vi "log analysis_gps.vi"() -> ()   [LabVIEW 2019] (continued)
0.4129,0.2981,0.5511,0.1100,0.0931,0.0771,0.1575,0.1588,4.9163,0f000001,0*d9024070\n\t", "INSPVAXA,USB3,0,48.5,FINESTEERING,2107,281880.250,02000000,471d,15824;INS_ALIGNMENT_COMPLETE,INS_RTKFIXED,37.37117348165,126.72305623679,7.9838,22.3000,-0.0959,0.2852,0.0145,-0.523517116,0.173445039,107.625224225,0.4131,0.2981,0.5507,0.1100,0.0932,0.0771,0.1574,0.1588,4.9179,0f000001,0*6bf7a559\n\t", "INSPVAXA,USB3,0,48.5,FINESTEERING,2107,281880.750,02000000,471d,15824;INS_ALIGNMENT_COMPLETE,INS_RTKFIXED,37.37117294431,126.72305789660,7.9831,22.3000,-0.0852,0.2698,0.0141,-0.555772515,0.079408991,107.669635072,0.4131,0.2981,0.5507,0.1100,0.0932,0.0771,0.1574,0.1588,4.9179,0f000001,0*1742ce26\n\t", "INSPVAXA,USB3,0,47.5,FINESTEERING,2107,281881.250,02000000,471d,15824;INS_ALIGNMENT_COMPLETE,INS_RTKFIXED,37.37117244492,126.72305941240,7.9826,22.3000,-0.0757,0.2574,0.0112,-0.499737353,0.074053137,107.349848920,0.4135,0.2983,0.5505,0.1102,0.0933,0.0771,0.1574,0.1588,4.9194,0f000001,0*402f3f2b\n\t", "INSPVAXA,USB3,0,47.5,FINESTEERING,2107,281881.750,02000000,471d,15824;INS_ALIGNMENT_COMPLETE,INS_RTKFIXED,37.37117196738,126.72306091172,7.9831,22.3000,-0.0783,0.2660,0.0186,-0.416436951,0.088853428,106.696307007,0.4135,0.2983,0.5505,0.1102,0.0933,0.0771,0.1574,0.1588,4.9194,0f000001,0*620f9249\n\t", "INSPVAXA,USB3,0,44.5,FINESTEERING,2107,281882.250,02000000,471d,15824;INS_ALIGNMENT_COMPLETE,INS_RTKFIXED,37.37117150853,126.72306241559,7.9850,22.3000,-0.0608,0.2451,0.0066,-0.406550409,0.024677772,105.806071956,0.4138,0.2984,0.5505,0.1102,0.0933,0.0771,0.1573,0.1588,4.9208,0f000001,0*20d266fd\n\t", "INSPVAXA,USB3,0,46.5,FINESTEERING,2107,281883.250,02000000,471d,15824;INS_ALIGNMENT_COMPLETE,INS_RTKFIXED,37.37117067641,126.72306545358,7.9876,22.3000,-0.0777,0.2473,0.0004,-0.446761173,0.141959315,103.301752998,0.4139,0.2985,0.5503,0.1102,0.0932,0.0771,0.1572,0.1587,4.9224,0f000001,0*34b690f3\n\t", "INSPVAXA,USB3,0,46.5,FINESTEERING,2107,281883.750,02000000,471d,15824;INS_ALIGNMENT_COMPLETE,INS_RTKFIXED,37.37117030441,126.72306700472,7.9899,22.3000,-0.0617,0.2696,0.0265,-0.542142026,0.246764373,102.057621753,0.4139,0.2985,0.5503,0.1102,0.0932,0.0771,0.1572,0.1587,4.9224,0f000001,0*016cab57\n\t", "INSPVAXA,USB3,0,48.0,FINESTEERING,2107,281884.750,02000000,471d,15824;INS_ALIGNMENT_COMPLETE,INS_RTKFIXED,37.37116962918,126.72307017450,7.9972,22.3000,-0.0537,0.2746,0.0133,-0.660873018,0.326948339,100.072587895,0.4139,0.2985,0.5502,0.1101,0.0931,0.0771,0.1571,0.1587,4.9240,0f000001,0*1475196f\n\t", "INSPVAXA,USB3,0,46.5,FINESTEERING,2107,281885.250,02000000,471d,15824;INS_ALIGNMENT_COMPLETE,INS_RTKFIXED,37.37116932974,126.72307175980,8.0003,22.3000,-0.0553,0.2834,0.0118,-0.680106492,0.432078155,99.489485657,0.4137,0.2985,0.5500,0.1099,0.0931,0.0771,0.1571,0.1587,4.9256,0f000001,0*384d6b59\n\t", "INSPVAXA,USB3,0,48.5,FINESTEERING,2107,281886.250,02000000,471d,15824;INS_ALIGNMENT_COMPLETE,INS_RTKFIXED,37.37116876559,126.72307497858,8.0043,22.3000,-0.0505,0.2700,0.0197,-0.630737523,0.236103622,98.774518000,0.4135,0.2984,0.5500,0.1099,0.0931,0.0771,0.1570,0.1587,4.9269,0f000001,0*06e1d073\n\t", "INSPVAXA,USB3,0,48.5,FINESTEERING,2107,281886.750,02000000,471d,15824;INS_ALIGNMENT_COMPLETE,INS_RTKFIXED,37.37116849518,126.72307655860,8.0058,22.3000,-0.0479,0.2894,0.0098,-0.729843639,0.253785173,98.685149837,0.4135,0.2984,0.5500,0.1099,0.0931,0.0771,0.1570,0.1587,4.9269,0f000001,0*6ed17162\n\t", "INSPVAXA,USB3,0,47.5,FINESTEERING,2107,281887.750,02000000,471d,15824;INS_ALIGNMENT_COMPLETE,INS_RTKFIXED,37.37116794085,126.72307975608,8.0103,22.3000,-0.0483,0.2817,0.0113,-0.853841864,0.188447476,98.810925200,0.4129,0.2983,0.5497,0.1100,0.0933,0.0771,0.1570,0.1587,4.9280,0f000001,0*b49a26d4\n\t", "INSPVAXA,USB3,0,50.0,FINESTEERING,2107,281888.250,02000000,471d,15824;INS_ALIGNMENT_COMPLETE,INS_RTKFIXED,37.37116766545,126.72308132013,8.0114,22.3000,-0.0457,0.2739,0.0034,-0.968854092,0.193025151,98.915996054,0.4125,0.2983,0.5497,0.1101,0.0935,0.0771,0.1571,0.1587,4.9288,0f000001,0*9b5c7e2f\n\t", "INSPVAXA,USB3,0,44.5,FINESTEERING,2107,281889.750,02000000,471d,15824;INS_ALIGNMENT_COMPLETE,INS_RTKFIXED,37.37116676559,126.72308604479,8.0182,22.3000,-0.0625,0.3054,0.0209,-0.972087805,-0.015873358,99.423505279,0.4122,0.2983,0.5496,0.1103,0.0935,0.0771,0.1571,0.1586,4.9293,0f000001,0*71ed46ba\n\t", "INSPVAXA,USB3,0,49.0,FINESTEERING,2107,281892.250,02000000,471d,15824;INS_ALIGNMENT_COMPLETE,INS_RTKFIXED,37.37116500965,126.72309429685,8.0266,22.3000,-0.0800,0.3032,0.0106,-1.000045816,-0.250485086,101.581647169,0.4117,0.2986,0.5496,0.1105,0.0935,0.0771,0.1571,0.1583,4.9290,0f000001,0*ebccc2b7\n\t", "INSPVAXA,USB3,0,49.0,FINESTEERING,2107,281892.750,02000000,471d,15824;INS_ALIGNMENT_COMPLETE,INS_RTKFIXED,37.37116464489,126.72309588370,8.0261,22.3000,-0.0746,0.2919,0.0013,-0.966505403,-0.074133262,102.355415882,0.4117,0.2986,0.5496,0.1105,0.0935,0.0771,0.1571,0.1583,4.9290,0f000001,0*e99d934b\n\t", "INSPVAXA,USB3,0,46.0,FINESTEERING,2107,281893.750,02000000,471d,15824;INS_ALIGNMENT_COMPLETE,INS_RTKFIXED,37.37116386545,126.72309901774,8.0239,22.3000,-0.0747,0.2810,0.0135,-0.903776454,0.116604665,103.770415844,0.4122,0.2987,0.5500,0.1103,0.0933,0.0771,0.1570,0.1582,4.9290,0f000001,0*419476b1\n\t", "INSPVAXA,USB3,0,46.0,FINESTEERING,2107,281895.250,02000000,471d,15824;INS_ALIGNMENT_COMPLETE,INS_RTKFIXED,37.37116255070,126.72310371548,8.0235,22.3000,-0.0988,0.2868,0.0058,-0.574989155,-0.045458111,105.108744593,0.4125,0.2988,0.5503,0.1099,0.0932,0.0771,0.1569,0.1580,4.9303,0f000001,0*d88c0d09\n\t", "INSPVAXA,USB3,0,48.5,FINESTEERING,2107,281911.800,02000000,471d,15824;INS_ALIGNMENT_COMPLETE,INS_RTKFIXED,37.37115003469,126.72315448526,8.0928,22.3000,-0.0862,0.2747,0.0289,-0.974037724,0.304621853,104.802649899,0.4114,0.2983,0.5457,0.1097,0.0931,0.0770,0.1565,0.1577,4.9486,0f000001,0*2c2c9bcb\n\t", "INSPVAXA,USB3,0,44.5,FINESTEERING,2107,281916.300,02000000,471d,15824;INS_ALIGNMENT_COMPLETE,INS_RTKFIXED,37.37114589383,126.72316794464,8.1130,22.3000,-0.1148,0.2616,0.0217,-1.148454264,0.358744068,107.173500933,0.4066,0.2960,0.5376,0.1089,0.0926,0.0764,0.1563,0.1575,4.9560,0f000001,0*04915923\n\t", "INSPVAXA,USB3,0,45.5,FINESTEERING,2107,281917.300,02000000,471d,15824;INS_ALIGNMENT_COMPLETE,INS_RTKFIXED,37.37114488879,126.72317107328,8.1169,22.3000,-0.1215,0.2812,0.0224,-1.106333570,0.024690310,107.280249927,0.4087,0.2971,0.5398,0.1096,0.0930,0.0767,0.1563,0.1576,4.9575,0f000001,0*9d9688b2\n\t", "INSPVAXA,USB3,0,48.5,FINESTEERING,2107,281918.800,02000000,471d,15824;INS_ALIGNMENT_COMPLETE,INS_RTKFIXED,37.37114346070,126.72317566723,8.1280,22.3000,-0.1055,0.2660,0.0189,-1.458385155,0.133384448,106.568583790,0.4097,0.2978,0.5415,0.1097,0.0931,0.0768,0.1562,0.1576,4.9589,0f000001,0*d5a698ac\n\t", "INSPVAXA,USB3,0,44.0,FINESTEERING,2107,281920.800,02000000,471d,15824;INS_ALIGNMENT_COMPLETE,INS_RTKFIXED,37.37114173890,126.72318175372,8.1382,22.3000,-0.1108,0.2593,0.0206,-1.441924072,0.214033238,104.164659813,0.4062,0.2959,0.5371,0.1088,0.0925,0.0764,0.1560,0.1575,4.9615,0f000001,0*96e1255f\n\t", "INSPVAXA,USB3,0,48.0,FINESTEERING,2107,281922.800,02000000,471d,15824;INS_ALIGNMENT_COMPLETE,INS_RTKFIXED,37.37114021696,126.72318792765,8.1435,22.3000,-0.0885,0.2559,0.0232,-1.379339371,0.280141219,102.369247536,0.4099,0.2977,0.5413,0.1094,0.0930,0.0768,0.1560,0.1575,4.9637,0f000001,0*69df9f1e\n\t", "INSPVAXA,USB3,0,48.0,FINESTEERING,2107,281923.800,02000000,471d,15824;INS_ALIGNMENT_COMPLETE,INS_RTKFIXED,37.37113946532,126.72319101111,8.1415,22.3000,-0.0919,0.2757,0.0244,-1.061632800,0.175078722,102.246819670,0.4052,0.2954,0.5349,0.1085,0.0923,0.0763,0.1558,0.1574,4.9646,0f000001,0*a7ce5637\n\t", "INSPVAXA,USB3,0,47.5,FINESTEERING,2107,281924.300,02000000,471d,15824;INS_ALIGNMENT_COMPLETE,INS_RTKFIXED,37.37113911142,126.72319252846,8.1410,22.3000,-0.0952,0.2671,0.0232,-1.111033615,0.347415537,102.293993552,0.4024,0.2943,0.5302,0.1081,0.0921,0.0760,0.1558,0.1574,4.9658,0f000001,0*38544010\n\t", "INSPVAXA,USB3,0,45.0,FINESTEERING,2107,281925.300,02000000,471d,15824;INS_ALIGNMENT_COMPLETE,INS_RTKFIXED,37.37113840523,126.72319556014,8.1418,22.3000,-0.0995,0.2785,0.0107,-1.061115952,0.585903196,102.432927019,0.4060,0.2962,0.5334,0.1089,0.0927,0.0764,0.1559,0.1575,4.9673,0f000001,0*3a408327\n\t", "INSPVAXA,USB3,0,47.0,FINESTEERING,2107,281926.800,02000000,471d,15824;INS_ALIGNMENT_COMPLETE,INS_RTKFIXED,37.37113727918,126.72320023038,8.1455,22.3000,-0.1010,0.2911,0.0183,-0.984134489,0.435250920,102.983735265,0.4086,0.2974,0.5364,0.1094,0.0930,0.0766,0.1559,0.1575,4.9689,0f000001,0*added2fa\n\t", "INSPVAXA,USB3,0,47.0,FINESTEERING,2107,281927.300,02000000,471d,15824;INS_ALIGNMENT_COMPLETE,INS_RTKFIXED,37.37113689419,126.72320185554,8.1485,22.3000,-0.1162,0.2988,0.0149,-1.006289928,0.413812859,103.207528579,0.4104,0.2981,0.5392,0.1096,0.0931,0.0768,0.1559,0.1575,4.9705,0f000001,0*f16ca07f\n\t", "INSPVAXA,USB3,0,48.5,FINESTEERING,2107,281928.300,02000000,471d,15824;INS_ALIGNMENT_COMPLETE,INS_RTKFIXED,37.37113611712,126.72320505771,8.1519,22.3000,-0.1090,0.2747,0.0204,-1.003980173,0.404401271,103.811290655,0.4113,0.2984,0.5414,0.1096,0.0931,0.0769,0.1559,0.1574,4.9721,0f000001,0*ce8a0efc\n\t", "INSPVAXA,USB3,0,47.0,FINESTEERING,2107,281929.300,02000000,471d,15824;INS_ALIGNMENT_COMPLETE,INS_RTKFIXED,37.37113535023,126.72320815380,8.1534,22.3000,-0.0933,0.2709,0.0146,-1.164082323,0.102490422,104.875233542,0.4118,0.2986,0.5433,0.1096,0.0930,0.0770,0.1559,0.1574,4.9735,0f000001,0*94f0b5d4\n\t", "INSPVAXA,USB3,0,49.0,FINESTEERING,2107,281930.300,02000000,471d,15824;INS_ALIGNMENT_COMPLETE,INS_RTKFIXED,37.37113452225,126.72321122959,8.1544,22.3000,-0.0922,0.2630,0.0022,-1.151432888,0.140260407,106.440387814,0.4107,0.2981,0.5430,0.1094,0.0928,0.0769,0.1559,0.1573,4.9747,0f000001,0*0b618f55\n\t", "INSPVAXA,USB3,0,46.5,FINESTEERING,2107,281931.300,02000000,471d,15824;INS_ALIGNMENT_COMPLETE,INS_RTKFIXED,37.37113361810,126.72321422448,8.1520,22.3000,-0.1052,0.2573,0.0056,-1.026339902,0.274196380,108.020288204,0.4094,0.2975,0.5419,0.1091,0.0927,0.0767,0.1558,0.1572,4.9758,0f000001,0*a4843e8d\n\t", "INSPVAXA,USB3,0,46.5,FINESTEERING,2107,281931.800,02000000,471d,15824;INS_ALIGNMENT_COMPLETE,INS_RTKFIXED,37.37113315554,126.72321571726,8.1497,22.3000,-0.1071,0.2546,0.0196,-1.189773358,0.228457398,108.723422614,0.4094,0.2975,0.5419,0.1091,0.0927,0.0767,0.1558,0.1572,4.9758,0f000001,0*2e0e4421\n\t", "INSPVAXA,USB3,0,46.5,FINESTEERING,2107,281932.800,02000000,471d,15824;INS_ALIGNMENT_COMPLETE,INS_RTKFIXED,37.37113218049,126.72321869652,8.1511,22.3000,-0.1122,0.2507,0.0244,-0.970343448,0.146977674,109.553158017,0.4088,0.2971,0.5408,0.1090,0.0926,0.0766,0.1558,0.1571,4.9770,0f000001,0*3507ce24\n\t", "INSPVAXA,USB3,0,46.5,FINESTEERING,2107,281933.300,02000000,471d,15824;INS_ALIGNMENT_COMPLETE,INS_RTKFIXED,37.37113167702,126.72322018624,8.1496,22.3000,-0.1082,0.2476,0.0112,-0.825942181,0.095830764,109.777034035,0.4078,0.2967,0.5396,0.1089,0.0928,0.0765,0.1558,0.1571,4.9781,0f000001,0*1bc6ffe3\n\t", "INSPVAXA,USB3,0,48.5,FINESTEERING,2107,281934.800,02000000,471d,15824;INS_ALIGNMENT_COMPLETE,INS_RTKFIXED,37.37113025084,126.72322449049,8.1432,22.3000,-0.1047,0.2449,0.0092,-0.950644980,-0.057069061,110.390138086,0.4095,0.2975,0.5414,0.1094,0.0930,0.0767,0.1558,0.1572,4.9791,0f000001,0*563aefdc\n\t", "INSPVAXA,USB3,0,46.5,FINESTEERING,2107,281935.300,02000000,471d,15824;INS_ALIGNMENT_COMPLETE,INS_RTKFIXED,37.37112977302,126.72322590337,8.1419,22.3000,-0.1049,0.2498,0.0104,-0.942926672,-0.039965742,110.562621563,0.4110,0.2981,0.5430,0.1097,0.0932,0.0768,0.1557,0.1572,4.9802,0f000001,0*75823065\n\t", "INSPVAXA,USB3,0,46.5,FINESTEERING,2107,281935.800,02000000,471d,15824;INS_ALIGNMENT_COMPLETE,INS_RTKFIXED,37.37112927929,126.72322735116,8.1404,22.3000,-0.1170,0.2611,0.0107,-1.050315231,0.030356412,110.657182537,0.4110,0.2981,0.5430,0.1097,0.0932,0.0768,0.1557,0.1572,4.9802,0f000001,0*518b09cb\n\t", "INSPVAXA,USB3,0,46.5,FINESTEERING,2107,281936.800,02000000,471d,15824;INS_ALIGNMENT_COMPLETE,INS_RTKFIXED,37.37112820521,126.72323038225,8.1394,22.3000,-0.1018,0.2637,0.0146,-1.057508289,0.307807352,110.761201411,0.4116,0.2984,0.5442,0.1099,0.0933,0.0768,0.1556,0.1572,4.9813,0f000001,0*af3d1803\n\t", "INSPVAXA,USB3,0,50.5,FINESTEERING,2107,281937.300,02000000,471d,15824;INS_ALIGNMENT_COMPLETE,INS_RTKFIXED,37.37112766751,126.72323189029,8.1401,22.3000,-0.1026,0.2581,0.0148,-1.068160739,0.434910636,110.781904334,0.4120,0.2986,0.5450,0.1099,0.0934,0.0769,0.1555,0.1571,4.9826,0f000001,0*c1896a38\n\t", "INSPVAXA,USB3,0,50.5,FINESTEERING,2107,281937.800,02000000,471d,15824;INS_ALIGNMENT_COMPLETE,INS_RTKFIXED,37.37112712976,126.72323340459,8.1402,22.3000,-0.1084,0.2649,0.0122,-1.080841395,0.445033455,110.675623077,0.4120,0.2986,0.5450,0.1099,0.0934,0.0769,0.1555,0.1571,4.9826,0f000001,0*491a3d94\n\t", "INSPVAXA,USB3,0,48.0,FINESTEERING,2107,281938.300,02000000,471d,15824;INS_ALIGNMENT_COMPLETE,INS_RTKFIXED,37.37112660699,126.72323489042,8.1401,22.3000,-0.1000,0.2525,0.0063,-1.085397063,0.578788009,110.287744750,0.4123,0.2988,0.5457,0.1100,0.0934,0.0769,0.1554,0.1571,4.9841,0f000001,0*2d3bbc15\n\t", "INSPVAXA,USB3,0,48.0,FINESTEERING,2107,281939.300,02000000,471d,15824;INS_ALIGNMENT_COMPLETE,INS_RTKFIXED,37.37112559001,126.72323792632,8.1403,22.3000,-0.1055,0.2758,-0.0006,-1.140987181,0.421010815,109.156991260,0.4088,0.2970,0.5408,0.1093,0.0930,0.0765,0.1552,0.1570,4.9858,0f000001,0*79dbeeff\n\t", "INSPVAXA,USB3,0,48.0,FINESTEERING,2107,281939.800,02000000,471d,15824;INS_ALIGNMENT_COMPLETE,INS_RTKFIXED,37.37112510387,126.72323945796,8.1419,22.3000,-0.1142,0.2830,0.0009,-1.038854179,0.260898620,108.398784803,0.4088,0.2970,0.5408,0.1093,0.0930,0.0765,0.1552,0.1570,4.9858,0f000001,0*5c0fede7\n\t", "INSPVAXA,USB3,0,46.0,FINESTEERING,2107,281940.800,02000000,471d,15824;INS_ALIGNMENT_COMPLETE,INS_RTKFIXED,37.37112421905,126.72324251509,8.1454,22.3000,-0.0917,0.2666,0.0165,-1.172718018,0.154583704,106.881501399,0.4059,0.2957,0.5358,0.1088,0.0926,0.0762,0.1550,0.1569,4.9872,0f000001,0*d9c0846d\n\t", "INSPVAXA,USB3,0,46.0,FINESTEERING,2107,281941.300,02000000,471d,15824;INS_ALIGNMENT_COMPLETE,INS_RTKFIXED,37.37112376695,126.72324410387,8.1465,22.3000,-0.0867,0.2640,0.0120,-1.227884261,0.058014022,106.288086050,0.4040,0.2951,0.5320,0.1086,0.0925,0.0760,0.1549,0.1568,4.9885,0f000001,0*dacbaea6\n\t", "INSPVAXA,USB3,0,46.0,FINESTEERING,2107,281941.800,02000000,471d,15824;INS_ALIGNMENT_COMPLETE,INS_RTKFIXED,37.37112332750,126.72324562221,8.1480,22.3000,-0.0872,0.2775,0.0087,-1.185427443,0.271965385,105.771989381,0.4040,0.2951,0.5320,0.1086,0.0925,0.0760,0.1549,0.1568,4.9885,0f000001,0*6fc02a4a\n\t", "INSPVAXA,USB3,0,48.0,FINESTEERING,2107,281942.300,02000000,471d,15824;INS_ALIGNMENT_COMPLETE,INS_RTKFIXED,37.37112291228,126.72324712545,8.1496,22.3000,-0.0882,0.2861,0.0099,-1.302160534,0.485080521,105.427907916,0.4030,0.2950,0.5294,0.1085,0.0925,0.0759,0.1549,0.1568,4.9897,0f000001,0*226a6453\n\t", "INSPVAXA,USB3,0,48.0,FINESTEERING,2107,281942.800,02000000,471d,15824;INS_ALIGNMENT_COMPLETE,INS_RTKFIXED,37.37112248759,126.72324869742,8.1506,22.3000,-0.0906,0.2829,0.0087,-1.416858091,0.320755573,105.114795692,0.4030,0.2950,0.5294,0.1085,0.0925,0.0759,0.1549,0.1568,4.9897,0f000001,0*d431e262\n\t", "DUALANTENNAHEADINGA,USB3,0,49.0,FINESTEERING,2107,281943.300,02000000,d426,15824;SOL_COMPUTED,NARROW_FLOAT,-1.000000000,117.129844666,-65.553436279,0.0,360.000000000,180.000000000,\"631T\",17,7,7,7,04,00,20,03*a0d5c722\n\t", "INSPVAXA,USB3,0,49.0,FINESTEERING,2107,281943.800,02000000,471d,15824;INS_ALIGNMENT_COMPLETE,INS_RTKFIXED,37.37112165725,126.72325176425,8.1526,22.3000,-0.0982,0.2663,0.0142,-1.467433834,0.522949098,104.939300217,0.4063,0.2966,0.5325,0.1091,0.0930,0.0763,0.1549,0.1569,4.9906,0f000001,0*8fab3056\n\t", "INSPVAXA,USB3,0,49.0,FINESTEERING,2107,281944.300,02000000,471d,15824;INS_ALIGNMENT_COMPLETE,INS_RTKFIXED,37.37112121835,126.72325329902,8.1549,22.3000,-0.0986,0.2706,0.0194,-1.288520157,0.440494920,104.991020886,0.4098,0.2978,0.5362,0.1096,0.0931,0.0766,0.1549,0.1570,4.9912,0f000001,0*9299408f\n\t", "INSPVAXA,USB3,0,49.0,FINESTEERING,2107,281944.800,02000000,471d,15824;INS_ALIGNMENT_COMPLETE,INS_RTKFIXED,37.37112078350,126.72325484675,8.1574,22.3000,-0.0973,0.2817,0.0195,-1.314361795,0.302961739,105.060294350,0.4098,0.2978,0.5362,0.1096,0.0931,0.0766,0.1549,0.1570,4.9912,0f000001,0*74de03e1\n\t", "INSPVAXA,USB3,0,50.5,FINESTEERING,2107,281945.300,02000000,471d,15824;INS_ALIGNMENT_COMPLETE,INS_RTKFIXED,37.37112035973,126.72325634532,8.1592,22.3000,-0.0947,0.2865,0.0177,-1.337666761,0.342742337,105.119539475,0.4078,0.2967,0.5345,0.1091,0.0927,0.0765,0.1549,0.1569,4.9918,0f000001,0*40c63c80\n\t", "DUALANTENNAHEADINGA,USB3,0,50.5,FINESTEERING,2107,281945.800,02000000,d426,15824;SOL_COMPUTED,NARROW_FLOAT,-1.000000000,110.210548401,-43.006103516,0.0,360.000000000,180.000000000,\"631T\",17,7,7,7,04,00,20,03*d65a3eb4\n\t", "DUALANTENNAHEADINGA,USB3,0,50.5,FINESTEERING,2107,281946.300,02000000,d426,15824;SOL_COMPUTED,NARROW_FLOAT,-1.000000000,136.716491699,-61.625274658,0.0,360.000000000,180.000000000,\"631T\",17,7,7,7,04,00,20,03*380a706b\n\t", "INSPVAXA,USB3,0,50.5,FINESTEERING,2107,281946.800,02000000,471d,15824;INS_ALIGNMENT_COMPLETE,INS_RTKFIXED,37.37111906801,126.72326090690,8.1646,22.3000,-0.0999,0.2885,0.0123,-1.416267608,0.329165481,105.354050291,0.4059,0.2956,0.5320,0.1087,0.0926,0.0762,0.1548,0.1568,4.9924,0f000001,0*28d47c8b\n\t", "INSPVAXA,USB3,0,45.5,FINESTEERING,2107,281947.300,02000000,471d,15824;INS_ALIGNMENT_COMPLETE,INS_RTKFIXED,37.37111863332,126.72326240814,8.1666,22.3000,-0.0961,0.2751,0.0203,-1.384816441,0.416422862,105.503918541,0.4041,0.2951,0.5298,0.1085,0.0924,0.0761,0.1549,0.1568,4.9930,0f000001,0*a10fe9f6\n\t", "INSPVAXA,USB3,0,45.5,FINESTEERING,2107,281947.800,02000000,471d,15824;INS_ALIGNMENT_COMPLETE,INS_RTKFIXED,37.37111818250,126.72326395318,8.1681,22.3000,-0.0954,0.2801,0.0190,-1.275593165,0.401297013,105.699844035,0.4041,0.2951,0.5298,0.1085,0.0924,0.0761,0.1549,0.1568,4.9930,0f000001,0*107534c5\n\t", "INSPVAXA,USB3,0,45.5,FINESTEERING,2107,281948.300,02000000,471d,15824;INS_ALIGNMENT_COMPLETE,INS_RTKFIXED,37.37111773045,126.72326549713,8.1704,22.3000,-0.0978,0.2931,0.0097,-1.304299318,0.393717319,105.933712093,0.4025,0.2945,0.5274,0.1083,0.0923,0.0760,0.1549,0.1567,4.9937,0f000001,0*f7f3e128\n\t", "DUALANTENNAHEADINGA,USB3,0,45.5,FINESTEERING,2107,281948.800,02000000,d426,15824;SOL_COMPUTED,NARROW_FLOAT,-1.000000000,181.763427734,-33.084808350,0.0,210.189346313,180.000000000,\"631T\",18,7,7,7,04,00,20,03*dd4d4ec1\n\t", "INSPVAXA,USB3,0,49.0,FINESTEERING,2107,281949.300,02000000,471d,15824;INS_ALIGNMENT_COMPLETE,INS_RTKFIXED,37.37111680262,126.72326852511,8.1763,22.3000,-0.0970,0.2807,0.0172,-1.183781176,0.416069138,106.325153596,0.4018,0.2942,0.5256,0.1083,0.0923,0.0759,0.1549,0.1566,4.9947,0f000001,0*47cb080a\n\t", "INSPVAXA,USB3,0,49.0,FINESTEERING,2107,281949.800,02000000,471d,15824;INS_ALIGNMENT_COMPLETE,INS_RTKFIXED,37.37111632001,126.72327008687,8.1784,22.3000,-0.0963,0.2886,0.0125,-1.143678600,0.359831061,106.512743553,0.4018,0.2942,0.5256,0.1083,0.0923,0.0759,0.1549,0.1566,4.9947,0f000001,0*07f750f1\n\t", "INSPVAXA,USB3,0,50.0,FINESTEERING,2107,281950.300,02000000,471d,15824;INS_ALIGNMENT_COMPLETE,INS_RTKFIXED,37.37111586312,126.72327158284,8.1822,22.3000,-0.0965,0.2844,0.0140,-1.158757889,0.473761966,106.723274256,0.4019,0.2945,0.5251,0.1083,0.0924,0.0759,0.1549,0.1566,4.9959,0f000001,0*c4604f56\n\t", "INSPVAXA,USB3,0,50.0,FINESTEERING,2107,281950.800,02000000,471d,15824;INS_ALIGNMENT_COMPLETE,INS_RTKFIXED,37.37111539537,126.72327311489,8.1870,22.3000,-0.0882,0.2799,0.0131,-1.063577950,0.631384742,106.921378709,0.4019,0.2945,0.5251,0.1083,0.0924,0.0759,0.1549,0.1566,4.9959,0f000001,0*182037fa\n\t", "DUALANTENNAHEADINGA,USB3,0,50.0,FINESTEERING,2107,281951.300,02000000,d426,15824;SOL_COMPUTED,NARROW_FLOAT,-1.000000000,139.470138550,7.252925396,0.0,360.000000000,180.000000000,\"631T\",16,7,7,7,04,00,20,03*6d09da6c\n\t", "INSPVAXA,USB3,0,50.0,FINESTEERING,2107,281951.800,02000000,471d,15824;INS_ALIGNMENT_COMPLETE,INS_RTKFIXED,37.37111448325,126.72327615215,8.1961,22.3000,-0.0961,0.2823,0.0155,-1.049815385,0.768292718,107.282719412,0.4015,0.2942,0.5235,0.1082,0.0922,0.0758,0.1549,0.1565,4.9974,0f000001,0*bdafe358\n\t", "INSPVAXA,USB3,0,49.0,FINESTEERING,2107,281952.300,02000000,471d,15824;INS_ALIGNMENT_COMPLETE,INS_RTKFIXED,37.37111402480,126.72327764482,8.2001,22.3000,-0.0943,0.2854,0.0221,-1.074547440,0.687119581,107.404842007,0.4042,0.2955,0.5263,0.1087,0.0925,0.0761,0.1549,0.1565,4.9990,0f000001,0*5102a955\n\t", "INSPVAXA,USB3,0,49.0,FINESTEERING,2107,281952.800,02000000,471d,15824;INS_ALIGNMENT_COMPLETE,INS_RTKFIXED,37.37111356857,126.72327910492,8.2050,22.3000,-0.0959,0.2790,0.0249,-1.146713469,0.626149533,107.488269865,0.4042,0.2955,0.5263,0.1087,0.0925,0.0761,0.1549,0.1565,4.9990,0f000001,0*a4159e63\n\t", "DUALANTENNAHEADINGA,USB3,0,51.5,FINESTEERING,2107,281953.300,02000000,d426,15824;SOL_COMPUTED,NARROW_FLOAT,-1.000000000,139.308395386,-63.930755615,0.0,360.000000000,171.725708008,\"631T\",19,7,7,7,04,00,20,03*aebc5255\n\t", "DUALANTENNAHEADINGA,USB3,0,51.5,FINESTEERING,2107,281953.800,02000000,d426,15824;SOL_COMPUTED,NARROW_FLOAT,-1.000000000,139.742797852,-63.902252197,0.0,360.000000000,171.789428711,\"631T\",17,7,7,7,04,00,20,03*2ba0ac3f\n\t", "INSPVAXA,USB3,0,49.5,FINESTEERING,2107,281954.300,02000000,471d,15824;INS_ALIGNMENT_COMPLETE,INS_RTKFIXED,37.37111212186,126.72328367661,8.2114,22.3000,-0.1061,0.2807,0.0084,-1.239615832,0.473328894,107.695107269,0.4028,0.2947,0.5241,0.1082,0.0921,0.0759,0.1549,0.1563,5.0021,0f000001,0*b68b8e11\n\t", "DUALANTENNAHEADINGA,USB3,0,49.5,FINESTEERING,2107,281954.800,02000000,d426,15824;SOL_COMPUTED,NARROW_FLOAT,-1.000000000,123.390388489,-57.995361328,0.0,360.000000000,180.000000000,\"631T\",16,7,7,7,04,00,20,03*cd5e4259\n\t", "DUALANTENNAHEADINGA,USB3,0,47.0,FINESTEERING,2107,281955.300,02000000,d426,15824;SOL_COMPUTED,NARROW_FLOAT,-1.000000000,132.237213135,-56.367187500,0.0,360.000000000,180.000000000,\"631T\",16,7,7,7,04,00,20,03*7928331b\n\t", "DUALANTENNAHEADINGA,USB3,0,47.0,FINESTEERING,2107,281955.800,02000000,d426,15824;SOL_COMPUTED,NARROW_FLOAT,-1.000000000,131.490509033,-56.782928467,0.0,360.000000000,180.000000000,\"631T\",17,7,7,7,04,00,20,03*bed209ba\n\t", "DUALANTENNAHEADINGA,USB3,0,47.0,FINESTEERING,2107,281956.300,02000000,d426,15824;SOL_COMPUTED,NARROW_FLOAT,-1.000000000,120.002708435,27.323427200,0.0,360.000000000,180.000000000,\"631T\",18,7,7,7,04,00,20,03*7e70b057\n\t", "INSPVAXA,USB3,0,47.0,FINESTEERING,2107,281956.800,02000000,471d,15824;INS_ALIGNMENT_COMPLETE,INS_RTKFIXED,37.37110977016,126.72329115727,8.2173,22.3000,-0.1059,0.2673,0.0082,-1.256961721,0.075845968,107.131843549,0.4006,0.2939,0.5214,0.1078,0.0919,0.0757,0.1548,0.1562,5.0048,0f000001,0*c3de906c\n\t", "INSPVAXA,USB3,0,49.0,FINESTEERING,2107,281957.300,02008000,471d,15824;INS_ALIGNMENT_COMPLETE,INS_RTKFIXED,37.37110932178,126.72329265930,8.2173,22.3000,-0.1030,0.2706,0.0074,-1.272872936,0.072348347,106.750132091,0.4007,0.2939,0.5208,0.1079,0.0919,0.0757,0.1548,0.1562,5.0062,0f000001,0*240beb48\n\t", "DUALANTENNAHEADINGA,USB3,0,49.0,FINESTEERING,2107,281957.800,02008000,d426,15824;SOL_COMPUTED,NARROW_FLOAT,-1.000000000,114.580795288,38.922153473,0.0,360.000000000,180.000000000,\"631T\",20,7,7,7,04,00,20,03*611330d6\n\t", "DUALANTENNAHEADINGA,USB3,0,49.5,FINESTEERING,2107,281958.300,02008000,d426,15824;SOL_COMPUTED,NARROW_FLOAT,-1.000000000,104.400451660,-50.100708008,0.0,360.000000000,180.000000000,\"631T\",21,7,7,7,04,00,20,03*9c19a85a\n\t", "DUALANTENNAHEADINGA,USB3,0,49.5,FINESTEERING,2107,281958.800,02008000,d426,15824;SOL_COMPUTED,NARROW_FLOAT,-1.000000000,106.192443848,-50.461669922,0.0,360.000000000,180.000000000,\"631T\",18,7,7,7,04,00,20,03*bd2737c2\n\t", "DUALANTENNAHEADINGA,USB3,0,47.5,FINESTEERING,2107,281959.300,02008000,d426,15824;SOL_COMPUTED,NARROW_FLOAT,-1.000000000,102.626930237,-53.845886230,0.0,360.000000000,180.000000000,\"631T\",18,7,7,7,04,00,20,03*cccf90f6\n\t", "DUALANTENNAHEADINGA,USB3,0,47.5,FINESTEERING,2107,281959.800,02008000,d426,15824;SOL_COMPUTED,NARROW_FLOAT,-1.000000000,103.518684387,-53.796081543,0.0,360.000000000,180.000000000,\"631T\",18,7,7,7,04,00,20,03*ff7adfc7\n\t", "INSPVAXA,USB3,0,50.0,FINESTEERING,2107,281960.300,02008000,471d,15824;INS_ALIGNMENT_COMPLETE,INS_RTKFIXED,37.37110689498,126.72330172800,8.2108,22.3000,-0.0740,0.2831,-0.0019,-1.608231411,0.368287071,104.214278774,0.4044,0.2959,0.5251,0.1086,0.0926,0.0761,0.1548,0.1563,5.0100,0f000001,0*1846b4aa\n\t", "INSPVAXA,USB3,0,50.0,FINESTEERING,2107,281960.800,02008000,471d,15824;INS_ALIGNMENT_COMPLETE,INS_RTKFIXED,37.37110653498,126.72330326832,8.2098,22.3000,-0.0639,0.2787,-0.0006,-1.592412104,0.419958697,103.937219008,0.4044,0.2959,0.5251,0.1086,0.0926,0.0761,0.1548,0.1563,5.0100,0f000001,0*83162285\n\t", "DUALANTENNAHEADINGA,USB3,0,46.5,FINESTEERING,2107,281961.300,02000000,d426,15824;SOL_COMPUTED,NARROW_FLOAT,-1.000000000,70.830032349,48.509868622,0.0,212.044555664,180.000000000,\"631T\",22,7,7,7,04,00,20,03*23813865\n\t", "DUALANTENNAHEADINGA,USB3,0,46.5,FINESTEERING,2107,281961.800,02000000,d426,15824;SOL_COMPUTED,NARROW_FLOAT,-1.000000000,72.091743469,46.579227448,0.0,218.795516968,180.000000000,\"631T\",20,7,7,7,04,00,20,03*2a3a9c35\n\t", "DUALANTENNAHEADINGA,USB3,0,46.5,FINESTEERING,2107,281962.300,02000000,d426,15824;SOL_COMPUTED,NARROW_FLOAT,-1.000000000,79.598190308,38.491451263,0.0,329.037414551,180.000000000,\"631T\",18,7,7,7,04,00,20,03*3c555fcd\n\t", "DUALANTENNAHEADINGA,USB3,0,46.5,FINESTEERING,2107,281962.800,02000000,d426,15824;SOL_COMPUTED,NARROW_FLOAT,-1.000000000,80.204544067,39.740882874,0.0,333.658050537,180.000000000,\"631T\",20,7,7,7,04,00,20,03*9ccf4ae9\n\t", "DUALANTENNAHEADINGA,USB3,0,45.5,FINESTEERING,2107,281963.300,02000000,d426,15824;SOL_COMPUTED,NARROW_FLOAT,-1.000000000,98.344001770,31.903175354,0.0,360.000000000,180.000000000,\"631T\",20,7,7,7,04,00,20,03*850b3b79\n\t", "DUALANTENNAHEADINGA,USB3,0,45.5,FINESTEERING,2107,281963.800,02000000,d426,15824;SOL_COMPUTED,NARROW_FLOAT,-1.000000000,99.070640564,30.000068665,0.0,360.000000000,180.000000000,\"631T\",18,7,7,7,04,00,20,03*27e895e1\n\t", "DUALANTENNAHEADINGA,USB3,0,47.5,FINESTEERING,2107,281964.300,02008000,d426,15824;SOL_COMPUTED,L1_FLOAT,-1.000000000,124.915382385,72.187736511,0.0,360.000000000,180.000000000,\"631T\",18,7,7,7,04,00,20,02*ef46fcdf\n\t", "DUALANTENNAHEADINGA,USB3,0,47.5,FINESTEERING,2107,281964.800,02008000,d426,15824;SOL_COMPUTED,L1_FLOAT,-1.000000000,123.601234436,72.153076172,0.0,360.000000000,180.000000000,\"631T\",20,7,7,7,04,00,20,03*2f9fd869\n\t", "DUALANTENNAHEADINGA,USB3,0,49.0,FINESTEERING,2107,281965.300,02008000,d426,15824;SOL_COMPUTED,NARROW_FLOAT,-1.000000000,138.902404785,50.477355957,0.0,360.000000000,180.000000000,\"631T\",21,7,7,7,04,00,20,03*697ae526\n\t", "DUALANTENNAHEADINGA,USB3,0,49.0,FINESTEERING,2107,281965.800,02008000,d426,15824;SOL_COMPUTED,NARROW_FLOAT,-1.000000000,141.790161133,47.706295013,0.0,360.000000000,180.000000000,\"631T\",19,7,7,7,04,00,20,03*80dc72b9\n\t", "DUALANTENNAHEADINGA,USB3,0,48.5,FINESTEERING,2107,281966.300,02008000,d426,15824;SOL_COMPUTED,NARROW_FLOAT,-1.000000000,166.037078857,-7.414306641,0.0,293.067352295,180.000000000,\"631T\",18,7,7,7,04,00,20,03*b88985fa\n\t", "DUALANTENNAHEADINGA,USB3,0,48.5,FINESTEERING,2107,281966.800,02008000,d426,15824;SOL_COMPUTED,NARROW_FLOAT,-1.000000000,165.893447876,-6.919708252,0.0,296.453521729,180.000000000,\"631T\",17,7,7,7,04,00,20,03*8e2fbaf6\n\t", "DUALANTENNAHEADINGA,USB3,0,48.5,FINESTEERING,2107,281967.300,02008000,d426,15824;SOL_COMPUTED,NARROW_FLOAT,-1.000000000,160.223464966,16.144151688,0.0,238.524597168,180.000000000,\"631T\",17,9,9,9,04,00,20,23*6b3012d0\n\t", "DUALANTENNAHEADINGA,USB3,0,48.5,FINESTEERING,2107,281967.800,02008000,d426,15824;SOL_COMPUTED,NARROW_FLOAT,-1.000000000,161.228576660,12.383532524,0.0,230.067184448,180.000000000,\"631T\",17,9,9,9,04,00,20,23*e747bf89\n\t", "DUALANTENNAHEADINGA,USB3,0,48.5,FINESTEERING,2107,281968.300,02000000,d426,15824;SOL_COMPUTED,NARROW_FLOAT,-1.000000000,166.146408081,14.704567909,0.0,156.659332275,180.000000000,\"631T\",17,9,9,9,04,00,20,23*68c6ea3a\n\t", "DUALANTENNAHEADINGA,USB3,0,48.5,FINESTEERING,2107,281968.800,02000000,d426,15824;SOL_COMPUTED,NARROW_FLOAT,-1.000000000,165.495330811,15.543543816,0.0,158.767318726,180.000000000,\"631T\",20,9,9,9,04,00,20,23*d314ab6c\n\t", "DUALANTENNAHEADINGA,USB3,0,49.0,FINESTEERING,2107,281969.300,02000000,d426,15824;SOL_COMPUTED,NARROW_FLOAT,-1.000000000,139.943130493,-43.141418457,0.0,292.614349365,180.000000000,\"631T\",18,9,9,9,04,00,20,23*245444fd\n\t", "DUALANTENNAHEADINGA,USB3,0,49.0,FINESTEERING,2107,281969.800,02000000,d426,15824;SOL_COMPUTED,NARROW_FLOAT,-1.000000000,140.197708130,-42.675354004,0.0,291.665954590,180.000000000,\"631T\",18,9,9,9,04,00,20,23*76897fdf\n\t", "DUALANTENNAHEADINGA,USB3,0,47.0,FINESTEERING,2107,281970.300,02000000,d426,15824;SOL_COMPUTED,NARROW_FLOAT,-1.000000000,136.818527222,-33.589324951,0.0,360.000000000,180.000000000,\"631T\",19,9,9,9,04,00,20,23*7b126b36\n\t", "DUALANTENNAHEADINGA,USB3,0,47.0,FINESTEERING,2107,281970.800,02000000,d426,15824;SOL_COMPUTED,NARROW_FLOAT,-1.000000000,136.650482178,-33.009735107,0.0,360.000000000,180.000000000,\"631T\",18,9,9,9,04,00,20,23*68bce87c\n\t", "DUALANTENNAHEADINGA,USB3,0,45.5,FINESTEERING,2107,281971.300,02000000,d426,15824;SOL_COMPUTED,NARROW_FLOAT,-1.000000000,137.123779297,-38.778259277,0.0,360.000000000,180.000000000,\"631T\",18,9,9,9,04,00,20,23*afd68441\n\t", "DUALANTENNAHEADINGA,USB3,0,45.5,FINESTEERING,2107,281971.800,02000000,d426,15824;SOL_COMPUTED,NARROW_FLOAT,-1.000000000,138.481918335,-40.903717041,0.0,360.000000000,180.000000000,\"631T\",17,7,7,7,04,00,20,03*998ba3b4\n\t", "DUALANTENNAHEADINGA,USB3,0,48.5,FINESTEERING,2107,281972.300,02000000,d426,15824;SOL_COMPUTED,NARROW_FLOAT,-1.000000000,122.800582886,-18.535125732,0.0,360.000000000,180.000000000,\"631T\",18,7,7,7,04,00,20,03*a3dfc53a\n\t", "DUALANTENNAHEADINGA,USB3,0,48.5,FINESTEERING,2107,281972.800,02000000,d426,15824;SOL_COMPUTED,NARROW_FLOAT,-1.000000000,124.024436951,-18.181030273,0.0,360.000000000,180.000000000,\"631T\",19,7,7,7,04,00,20,03*7aaae106\n\t", "DUALANTENNAHEADINGA,USB3,0,47.5,FINESTEERING,2107,281973.300,02000000,d426,15824;SOL_COMPUTED,NARROW_FLOAT,-1.000000000,122.042884827,-22.737487793,0.0,360.000000000,180.000000000,\"631T\",19,7,7,7,04,00,20,03*1f55fb10\n\t", "DUALANTENNAHEADINGA,USB3,0,47.5,FINESTEERING,2107,281973.800,02000000,d426,15824;SOL_COMPUTED,NARROW_FLOAT,-1.000000000,123.718307495,-22.855773926,0.0,360.000000000,180.000000000,\"631T\",19,7,7,7,04,00,20,03*d5b1223e\n\t", "DUALANTENNAHEADINGA,USB3,0,47.5,FINESTEERING,2107,281974.300,02000000,d426,15824;SOL_COMPUTED,NARROW_FLOAT,-1.000000000,126.303939819,-25.588958740,0.0,360.000000000,180.000000000,\"631T\",20,7,7,7,04,00,20,03*39a380db\n\t", "INSPVAXA,USB3,0,49.5,FINESTEERING,2107,281977.350,02008000,471d,15824;INS_ALIGNMENT_COMPLETE,INS_RTKFIXED,37.37109525402,126.72334121062,8.2543,22.3000,-0.1170,0.2421,0.0133,-1.435832187,0.337185774,113.410271664,0.3981,0.2933,0.5166,0.1081,0.0923,0.0755,0.1541,0.1553,4.9775,0f000001,0*5c2d119f\n\t", "DUALANTENNAHEADINGA,USB3,0,47.5,FINESTEERING,2107,281978.800,02008000,d426,15824;SOL_COMPUTED,NARROW_FLOAT,-1.000000000,98.850494385,15.051933289,0.0,360.000000000,180.000000000,\"631T\",20,7,7,7,04,00,20,03*20b61e65\n\t", "INSPVAXA,USB3,0,49.0,FINESTEERING,2107,281979.350,02008000,471d,15824;INS_ALIGNMENT_COMPLETE,INS_RTKFIXED,37.37109277757,126.72334695019,8.2625,22.3000,-0.1363,0.2541,0.0099,-1.083954396,0.543239164,111.989343761,0.3985,0.2934,0.5159,0.1083,0.0925,0.0755,0.1539,0.1552,4.9769,0f000001,0*5af8ae3d\n\t", "INSPVAXA,USB3,0,49.0,FINESTEERING,2107,281979.850,02008000,471d,15824;INS_ALIGNMENT_COMPLETE,INS_RTKFIXED,37.37109223488,126.72334834985,8.2645,22.3000,-0.1140,0.2510,0.0288,-1.130767744,0.597027739,110.592195970,0.3985,0.2934,0.5159,0.1083,0.0925,0.0755,0.1539,0.1552,4.9769,0f000001,0*c15e5176\n\t", "INSPVAXA,USB3,0,47.5,FINESTEERING,2107,281980.350,02008000,471d,15824;INS_ALIGNMENT_COMPLETE,INS_RTKFIXED,37.37109170650,126.72334980236,8.2673,22.3000,-0.1001,0.2682,0.0069,-1.052775412,0.394834904,108.778696674,0.3992,0.2936,0.5159,0.1082,0.0924,0.0755,0.1537,0.1552,4.9781,0f000001,0*7c12e27f\n\t", "DUALANTENNAHEADINGA,USB3,0,47.5,FINESTEERING,2107,281981.800,02000000,d426,15824;SOL_COMPUTED,NARROW_FLOAT,-1.000000000,85.660850525,58.330966949,0.0,360.000000000,180.000000000,\"631T\",21,7,7,7,04,00,20,03*4d1d89aa\n\t", "DUALANTENNAHEADINGA,USB3,0,50.0,FINESTEERING,2107,281982.300,02000000,d426,15824;SOL_COMPUTED,NARROW_FLOAT,-1.000000000,91.491950989,60.466197968,0.0,360.000000000,180.000000000,\"631T\",20,7,7,7,04,00,20,03*c36635f4\n\t", "INSPVAXA,USB3,0,50.0,FINESTEERING,2107,281982.850,02000000,471d,15824;INS_ALIGNMENT_COMPLETE,INS_RTKFIXED,37.37108972334,126.72335727408,8.2765,22.3000,-0.0719,0.2745,0.0019,-0.882780999,0.621145349,100.706035847,0.4014,0.2941,0.5170,0.1080,0.0922,0.0756,0.1534,0.1551,4.9808,0f000001,0*8125501e\n\t", "INSPVAXA,USB3,0,50.0,FINESTEERING,2107,281983.350,02000000,471d,15824;INS_ALIGNMENT_COMPLETE,INS_RTKFIXED,37.37108941060,126.72335884904,8.2775,22.3000,-0.0682,0.2732,0.0044,-0.923445241,0.570606405,99.817736396,0.4009,0.2937,0.5167,0.1077,0.0921,0.0755,0.1533,0.1550,4.9813,0f000001,0*fb321f29\n\t", "DUALANTENNAHEADINGA,USB3,0,50.0,FINESTEERING,2107,281983.800,02000000,d426,15824;SOL_COMPUTED,NARROW_FLOAT,-1.000000000,171.677200317,69.382904053,0.0,261.160797119,118.765472412,\"631T\",16,7,7,7,04,00,20,03*68664d6e\n\t", "DUALANTENNAHEADINGA,USB3,0,49.0,FINESTEERING,2107,281984.800,02000000,d426,15824;SOL_COMPUTED,NARROW_FLOAT,-1.000000000,180.068710327,69.173255920,0.0,191.709030151,111.731857300,\"631T\",18,7,7,7,04,00,20,03*3faf2cde\n\t", "INSPVAXA,USB3,0,51.5,FINESTEERING,2107,281985.350,02000000,471d,15824;INS_ALIGNMENT_COMPLETE,INS_RTKFIXED,37.37108883978,126.72336045763,8.2740,22.3000,-0.0197,0.0054,0.0046,-0.783405555,0.390647361,99.517937429,0.4021,0.2930,0.5155,0.1100,0.0923,0.0753,0.1532,0.1549,4.9767,0f000001,0*248bca7d\n\t", "INSPVAXA,USB3,0,51.5,FINESTEERING,2107,281985.850,02000000,471d,15824;INS_ALIGNMENT_COMPLETE,INS_RTKFIXED,37.37108879564,126.72336048903,8.2732,22.3000,-0.0176,0.0072,0.0041,-0.785106816,0.393235507,99.515755196,0.4021,0.2930,0.5155,0.1100,0.0923,0.0753,0.1532,0.1549,4.9767,0f000001,0*274b58cf\n\t", "INSPVAXA,USB3,0,48.0,FINESTEERING,2107,281986.350,02000000,471d,15824;INS_ALIGNMENT_COMPLETE,INS_RTKFIXED,37.37108876739,126.72336052169,8.2716,22.3000,-0.0165,0.0095,0.0036,-0.784401118,0.395223207,99.515202134,0.4035,0.2929,0.5152,0.1096,0.0926,0.0753,0.1533,0.1548,4.9684,0f000001,0*a346e64c\n\t", "INSPVAXA,USB3,0,48.0,FINESTEERING,2107,281986.850,02000000,471d,15824;INS_ALIGNMENT_COMPLETE,INS_RTKFIXED,37.37108874345,126.72336056234,8.2697,22.3000,-0.0165,0.0121,0.0038,-0.783492402,0.394489755,99.515268090,0.4035,0.2929,0.5152,0.1096,0.0926,0.0753,0.1533,0.1548,4.9684,0f000001,0*d15eefc4\n\t", "INSPVAXA,USB3,0,47.5,FINESTEERING,2107,281988.850,02000000,471d,15824;INS_ALIGNMENT_COMPLETE,INS_RTKFIXED,37.37108797326,126.72336627998,8.2767,22.3000,-0.0630,0.2990,0.0131,-1.082198945,0.183813421,99.716659847,0.4039,0.2931,0.5146,0.1091,0.0928,0.0753,0.1533,0.1544,4.9498,0f000001,0*73d74fed\n\t", "INSPVAXA,USB3,0,47.5,FINESTEERING,2107,281989.350,02000000,471d,15824;INS_ALIGNMENT_COMPLETE,INS_RTKFIXED,37.37108771760,126.72336784946,8.2786,22.3000,-0.0596,0.2938,0.0092,-0.873489656,0.138919963,99.763055093,0.4016,0.2938,0.5156,0.1102,0.0931,0.0754,0.1533,0.1542,4.9496,0f000001,0*cc44b012\n\t", "INSPVAXA,USB3,0,48.0,FINESTEERING,2107,281990.850,02000000,471d,15824;INS_ALIGNMENT_COMPLETE,INS_RTKFIXED,37.37108694002,126.72337277307,8.2855,22.3000,-0.0481,0.3030,0.0049,-0.965496149,0.214981023,98.709278858,0.4041,0.2964,0.5214,0.1116,0.0937,0.0758,0.1533,0.1541,4.9510,0f000001,0*3e871dfa\n\t", "INSPVAXA,USB3,0,49.5,FINESTEERING,2107,281991.350,02000000,471d,15824;INS_ALIGNMENT_COMPLETE,INS_RTKFIXED,37.37108669886,126.72337439108,8.2873,22.3000,-0.0502,0.3004,0.0017,-1.174650007,0.215279567,98.185602057,0.4065,0.2980,0.5270,0.1121,0.0939,0.0762,0.1533,0.1539,4.9506,0f000001,0*29bf6a14\n\t", "INSPVAXA,USB3,0,48.5,FINESTEERING,2107,281992.350,02008000,471d,15824;INS_ALIGNMENT_COMPLETE,INS_RTKFIXED,37.37108621097,126.72337762308,8.2906,22.3000,-0.0509,0.3067,0.0077,-1.111919380,0.301360235,97.469482841,0.4135,0.2993,0.5341,0.1130,0.0941,0.0766,0.1532,0.1538,4.9480,0f000001,0*f7c4fc4c\n\t", "INSPVAXA,USB3,0,48.5,FINESTEERING,2107,281992.850,02008000,471d,15824;INS_ALIGNMENT_COMPLETE,INS_RTKFIXED,37.37108597752,126.72337923306,8.2930,22.3000,-0.0486,0.3061,0.0133,-1.174980887,0.150326123,97.387759398,0.4135,0.2993,0.5341,0.1130,0.0941,0.0766,0.1532,0.1538,4.9480,0f000001,0*c1faa1b5\n\t", "INSPVAXA,USB3,0,46.0,FINESTEERING,2107,281993.350,02008000,471d,15824;INS_ALIGNMENT_COMPLETE,INS_RTKFIXED,37.37108573998,126.72338082832,8.2949,22.3000,-0.0500,0.2978,0.0061,-1.421543632,0.145972145,97.447075083,0.4166,0.2999,0.5394,0.1132,0.0941,0.0768,0.1531,0.1535,4.9437,0f000001,0*17ed31ac\n\t", "INSPVAXA,USB3,0,46.0,FINESTEERING,2107,281993.850,02008000,471d,15824;INS_ALIGNMENT_COMPLETE,INS_RTKFIXED,37.37108548434,126.72338234457,8.2959,22.3000,-0.0500,0.2833,0.0078,-1.457872405,0.272327462,97.575825981,0.4166,0.2999,0.5394,0.1132,0.0941,0.0768,0.1531,0.1535,4.9437,0f000001,0*5caa60c3\n\t", "INSPVAXA,USB3,0,49.0,FINESTEERING,2107,281994.850,02008000,471d,15824;INS_ALIGNMENT_COMPLETE,INS_RTKFIXED,37.37108494308,126.72338542204,8.3016,22.3000,-0.0524,0.2963,0.0111,-1.327091398,0.262905229,97.908015700,0.4162,0.2999,0.5423,0.1120,0.0939,0.0768,0.1530,0.1531,4.9380,0f000001,0*42f9b06f\n\t", "INSPVAXA,USB3,0,47.5,FINESTEERING,2107,281995.350,02008000,471d,15824;INS_ALIGNMENT_COMPLETE,INS_RTKFIXED,37.37108466032,126.72338706837,8.3039,22.3000,-0.0576,0.3333,-0.0065,-1.460342907,0.308573578,98.178770776,0.4137,0.2991,0.5422,0.1112,0.0936,0.0766,0.1529,0.1527,4.9332,0f000001,0*ae64a2a4\n\t", "INSPVAXA,USB3,0,47.5,FINESTEERING,2107,281995.850,02008000,471d,15824;INS_ALIGNMENT_COMPLETE,INS_RTKFIXED,37.37108438124,126.72338871075,8.3072,22.3000,-0.0531,0.3233,-0.0006,-1.819145416,0.336322767,98.552237530,0.4137,0.2991,0.5422,0.1112,0.0936,0.0766,0.1529,0.1527,4.9332,0f000001,0*cbb88409\n\t", "INSPVAXA,USB3,0,47.5,FINESTEERING,2107,281996.350,02000000,471d,15824;INS_ALIGNMENT_COMPLETE,INS_RTKFIXED,37.37108408170,126.72339032288,8.3123,22.3000,-0.0750,0.3139,0.0177,-1.695760628,0.287982482,99.034005489,0.4135,0.2988,0.5426,0.1109,0.0935,0.0765,0.1528,0.1525,4.9294,0f000001,0*c8ba75d6\n\t", "INSPVAXA,USB3,0,47.5,FINESTEERING,2107,281996.850,02000000,471d,15824;INS_ALIGNMENT_COMPLETE,INS_RTKFIXED,37.37108376936,126.72339189832,8.3173,22.3000,-0.0870,0.3015,0.0104,-1.544598209,0.423694709,99.865488428,0.4135,0.2988,0.5426,0.1109,0.0935,0.0765,0.1528,0.1525,4.9294,0f000001,0*decac9b0\n\t", "INSPVAXA,USB3,0,47.0,FINESTEERING,2107,281997.350,02000000,471d,15824;INS_ALIGNMENT_COMPLETE,INS_RTKFIXED,37.37108342179,126.72339342311,8.3197,22.3000,-0.0655,0.2686,0.0098,-1.474135417,0.714052944,100.935237660,0.4109,0.2981,0.5411,0.1099,0.0931,0.0764,0.1526,0.1523,4.9264,0f000001,0*027bf543\n\t", "INSPVAXA,USB3,0,47.0,FINESTEERING,2107,281997.850,02000000,471d,15824;INS_ALIGNMENT_COMPLETE,INS_RTKFIXED,37.37108303856,126.72339495769,8.3212,22.3000,-0.0845,0.2926,0.0185,-1.495781982,0.741465354,102.154050788,0.4109,0.2981,0.5411,0.1099,0.0931,0.0764,0.1526,0.1523,4.9264,0f000001,0*92cd812c\n\t", "DUALANTENNAHEADINGA,USB3,0,46.5,FINESTEERING,2107,281998.300,02000000,d426,15824;SOL_COMPUTED,NARROW_FLOAT,-1.000000000,172.084686279,54.228965759,0.0,275.366882324,180.000000000,\"631T\",18,9,9,9,04,00,20,23*6c4f8940\n\t", "INSPVAXA,USB3,0,46.5,FINESTEERING,2107,281998.850,02000000,471d,15824;INS_ALIGNMENT_COMPLETE,INS_RTKFIXED
